vi "Move to Point.vi"() -> ()   [LabVIEW 2020]
uses:
  Aerotech.lvlib
  Controller/Controller.lvclass
panel:
  in  "speed":dbl
  in  "XY Start":dbl[](array[numeric])
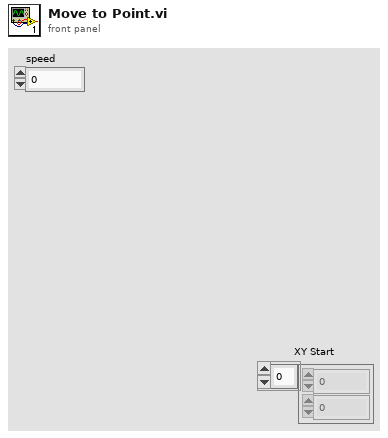
[diagram p1: front panel]
types:
  T1 = typedef "Controller.lvclass/Controllers.ctl" = cluster{"I-O.lvclass":refnum<class "I-O.lvclass">, "Dispenser.lvclass":refnum<class "Dispenser.lvclass">, "Gantry":refnum<k24>}
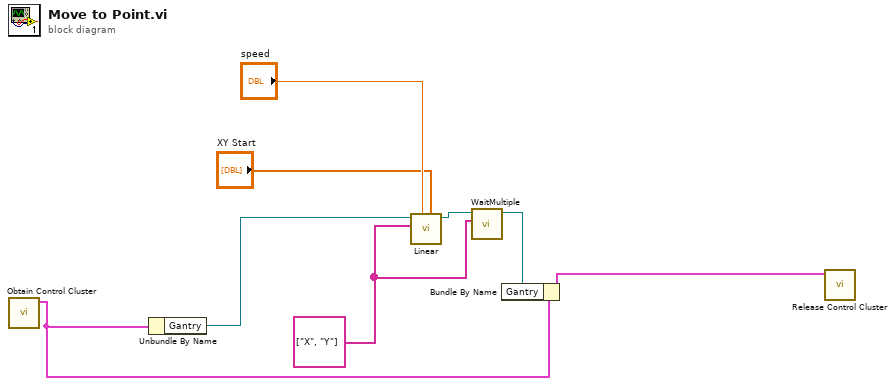
[diagram p0: block diagram]
diagram:
  w2 = string[] ["X", "Y"] ("axis names")
  n1 = call "Obtain Control Cluster.vi"() -> ("Control Out"=w5:T1)  [unwired: 11 in]
  n2 = Unbundle By Name(w5) -> ("Gantry"=w7:refnum<k24>)
  n3 = call "Linear.vi"("distances"="XY Start", "speed"="speed", "axis names"=w2, "controller in"=w7) -> ("controller out"=w3:refnum<k24>)  [unwired: 6 in, 1 out]
  n4 = call "WaitMultiple.vi"("axis names"=w2, "controller in"=w3) -> ("controller out"=w1:refnum<k24>)  [unwired: 7 in, 2 out]
  n5 = Bundle By Name(cluster=w5, "Gantry"=w1) -> (w4:T1)
  n6 = call "Release Control Cluster.vi"("output cluster"=w4) -> ()  [unwired: 11 in]
